vi "Read FPGA Session.vi"(8 "error in (no error)":errorcluster, 11 "ePAS in":refnum<class "ePAS.lvclass">) -> (0 "error out":errorcluster, 2 "Session Handle":T1, 3 "ePAS out":refnum<class "ePAS.lvclass">)   [LabVIEW 2015, in "ePAS Library.lvlib" / "ePAS.lvclass"]
uses:
  ePAS.lvclass
  <vilib>/MSR Consulting, LLC/ESF/Typedefs/Session Handle.ctl
  <vilib>/MSR Consulting, LLC/ESF/Session - Root.lvclass
  ePAS.lvclass/ePAS.ctl
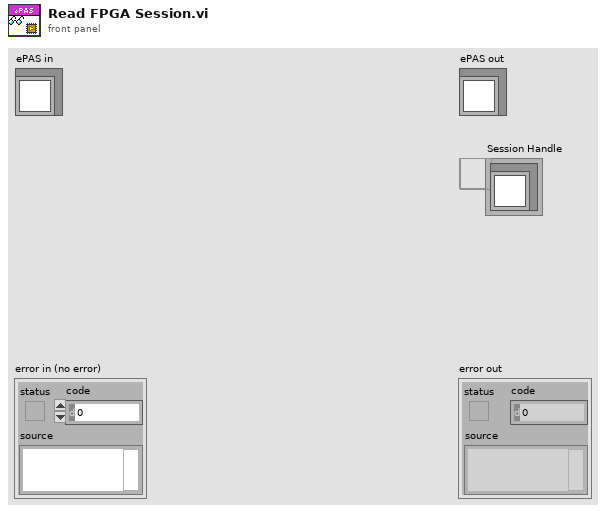
[diagram p1: front panel]
types:
  T1 = typedef "Session - Root.lvclass/Session Handle.ctl" = refnum<data-value>
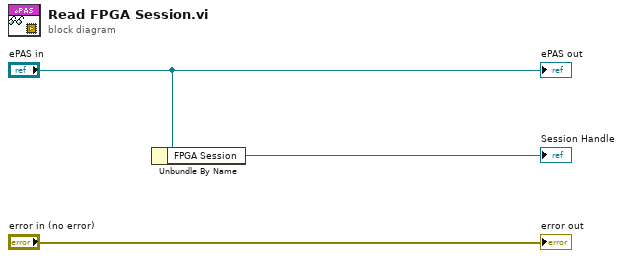
[diagram p0: block diagram]
diagram:
  n1 = Unbundle By Name("ePAS in") -> ("FPGA Session"=→"Session Handle":T1)
  "error out" <- "error in (no error)"
  "ePAS out" <- "ePAS in"
